vi "Find Group Sample Rate.vi"(8 "error in (no error)":errorcluster, 10 "Controls":T1[](array[typedef]) {"Data Type" format="%.0x"}, 11 "group":string) -> (0 "error out":errorcluster, 1 "Rate":dbl, 2 "Register":T1={"Name"="", "Data Type"=enum."<Null>", "Default Value"=variant(dbl 0.0)} {"Data Type" format="%.0x"})   [LabVIEW 2015, in "Fuel Injector Analysis Addon System Explorer.lvlib"]
uses:
  Fuel Injector Analysis Addon System Explorer.lvlib
  Shared/Types/Register.Info.ctl
  Shared/Types/FPGA Data Types.ctl
  Shared/Fuel Injector Analysis Addon Shared.lvlib
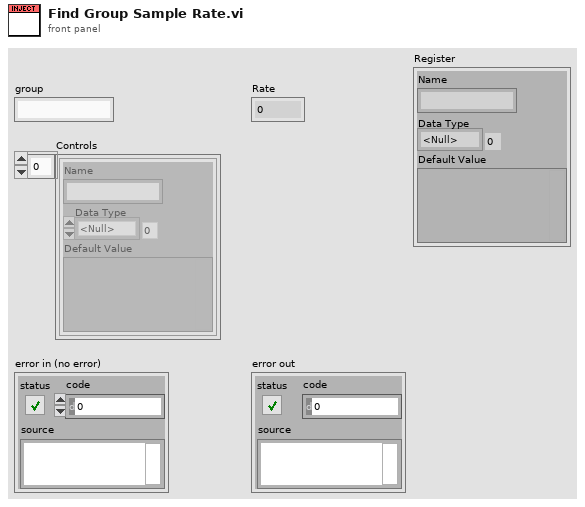
[diagram p1: front panel]
types:
  T1 = typedef "Fuel Injector Analysis Addon Shared.lvlib/Register.Info.ctl" = cluster{"Name":string, "Data Type":T2, "Default Value":variant}
  T2 = typedef "Fuel Injector Analysis Addon Shared.lvlib/FPGA Data Types.ctl" = enum8{"<Null>", "Injector.Core.Setting", "Injector.Global.Setting", "Injector.Mux.Setting", "Injector.Timing"}
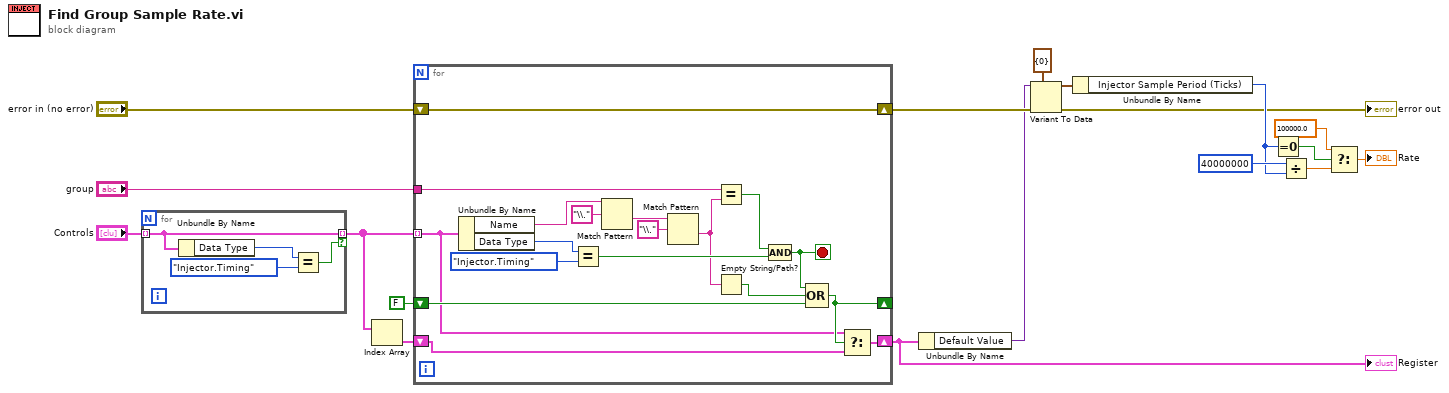
[diagram p0: block diagram]
diagram:
  n1 = for {
    tunnel: "Controls" -> [w20] mode=indexing
    tunnel: [w20] -> w2 mode=indexing if=w19
    n2 = Unbundle By Name(w20) -> ("Data Type"=w22:T2)
    n3 = Equal?(x=w22, y=FPGA_Data_Types."Injector.Timing") -> (x = y?=w19:bool)
  }
  n4 = Index Array(array=w2) -> (element=w1:T1)  [unwired: 1 in]
  n5 = for {
    tunnel: w2 -> [w25] mode=indexing
    shift-right: [w24] -> w7
    shift-left: "error in (no error)" -> [w24]
    tunnel: "group" -> [w37]
    shift-right: [w28] -> _
    shift-left: FALSE -> [w29]
    shift-right: [w26] -> w8
    shift-left: w1 -> [w27]
    stop <- w23 stop-if-true
    n6 = Unbundle By Name(w25) -> ("Name"=w32:string, "Data Type"=w40:T2)
    n7 = Equal?(x=w40, y=FPGA_Data_Types."Injector.Timing") -> (x = y?=w38:bool)
    n8 = Match Pattern(string=w32, regular expression="\\.") -> (after substring=w35:string)  [unwired: 1 in, 3 out]
    n9 = Match Pattern(string=w35, regular expression="\\.") -> (after substring=w31:string)  [unwired: 1 in, 3 out]
    n10 = Equal?(x=w37, y=w31) -> (x = y?=w36:bool)
    n11 = Empty String/Path?(string/path=w31) -> (empty?=w30:bool)
    n12 = Compound Arithmetic op=AND(w36, w38) -> (w23:bool)
    n13 = Compound Arithmetic op=OR(w23, w30, w29) -> (w28:bool)
    n14 = Select(t=w25, s=w28, f=w27) -> (s? t:f=w26:T1)
  }
  "Register" <- w8
  n15 = Unbundle By Name(w8) -> ("Default Value"=w6:variant)
  n16 = Variant To Data(error in=w7, type=cluster{"Injector Sample Period (Ticks)":u32} {"Injector Sample Period (Ticks)"=0} ("Injector.Timing"), Variant=w6) -> (data=w13:cluster{"Injector Sample Period (Ticks)":u32}, error out=→"error out":errorcluster)
  n17 = Unbundle By Name(w13) -> ("Injector Sample Period (Ticks)"=w12:u32)
  n18 = Equal To 0?(x=w12) -> (x = 0?=w11:bool)
  n19 = Divide(x=u32 40000000, y=w12) -> (x/y=w9:dbl)
  n20 = Select(t=100000.0, s=w11, f=w9) -> (s? t:f=→"Rate":dbl)
